vi "Set Pin.vi"(0 "Arduino in":refnum<class "Arduino.lvclass">, 5 "VISA resource name":refnum<visa-resource-name>, 7 "Pin":u8, 9 "Pin State":bool, 11 "error in (no error)":errorcluster) -> (4 "Arduino out":refnum<class "Arduino.lvclass">, 6 "VISA resource name 2":refnum<visa-resource-name>, 15 "error out":errorcluster)   [LabVIEW 2020, in "Arduino.lvclass"]
uses:
  Arduino.lvclass
  Abstract/Serial Device/Serial Device.lvclass
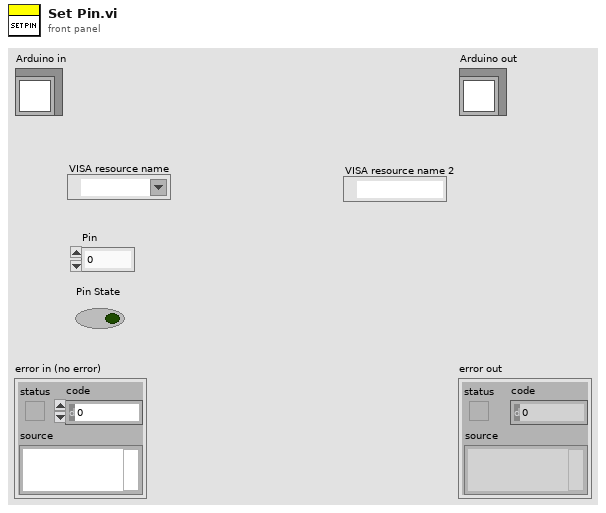
[diagram p1: front panel]
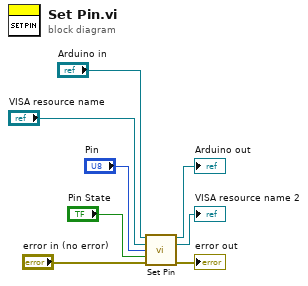
[diagram p0: block diagram]
diagram:
  n1 = call-parent "Set Pin.vi"("Serial Device in"="Arduino in", "VISA resource name"="VISA resource name", "Pin"="Pin", "Pin State"="Pin State", "error in (no error)"="error in (no error)") -> ("Serial Device out"=→"Arduino out":refnum<class "Arduino.lvclass">, "VISA resource name 2"=→"VISA resource name 2":refnum<visa-resource-name>, "error out"=→"error out":errorcluster)  [unwired: 8 in]
